vi "ClimbAverages.vi"(0 "String in":string) -> (7 "String out":string)   [LabVIEW 2015]
uses:
  Global Data.vi
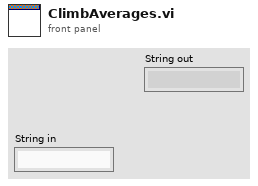
[diagram p1: front panel]
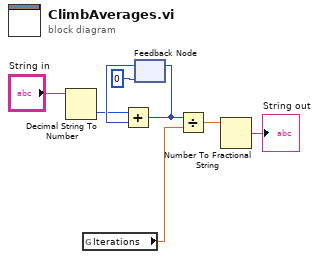
[diagram p0: block diagram]
diagram:
  n1 = Decimal String To Number(string="String in") -> (number=w5:i32)  [unwired: 2 in, 1 out]
  n2 = global read "Global Data.vi" "Iterations"() -> (w1:ext)
  n3 = feedback #1(0) -> (w7:i32)
  n4 = Add(x=w5, y=w7) -> (x+y=w6:i32)
  n5 = feedback-in #1(w6) -> ()
  n6 = Divide(x=w6, y=w1) -> (x/y=w3:ext)
  n7 = Number To Fractional String(number=w3) -> (F-format string=→"String out":string)  [unwired: 3 in]
